vi "CPP_WhiteNoiseGenerator.vi"() -> ()   [LabVIEW 2012]
uses:
  <vilib>/sound2/lvsound2.llb/Sound Data Format.ctl
  <vilib>/sound2/lvsound2.llb/Sampling Mode.ctl
  <vilib>/Analysis/3filter.llb/Filter Passband Type.ctl
  Globals/Meas_global.vi
  Plug in sub vis/CPP_TubingCompensation/WhiteNoise/WhiteNoiseGlobal.vi
  <vilib>/Analysis/3filter.llb/Butterworth Filter (DBL).vi
  <vilib>/sound2/lvsound2.llb/Sound Output Write (DBL Single).vi
  <vilib>/measure/NI_MABase.lvlib
  <vilib>/Analysis/NI_AALBase.lvlib
panel:
  in  "Device ID":u32
  in  "Amplitude":dbl=1.0
  in  "Cutoff (Hz)":dbl=1000.0
  in  "Overproduce":dbl=1.2
  out "Duration (s)":dbl=16.0
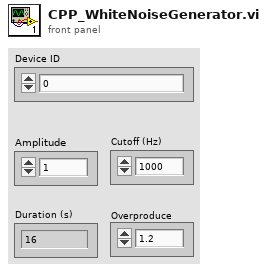
[diagram p1: front panel]
types:
  T1 = typedef "Post_Process.ctl" = enum16{"Take New Data", "Post Process Raw Data File"}
  T2 = typedef "NI_AALBase.lvlib/Filter Passband Type.ctl" = enum32{"Lowpass", "Highpass", "Bandpass", "Bandstop"}
  T3 = typedef "Sampling Mode.ctl" = i32
  T4 = typedef "Sound Data Format.ctl" = cluster{"sample rate (S/s)":dbl, "number of channels":i32, "bits per sample":i32}
  T5 = typedef "Sound Output Task ID.ctl" = u32
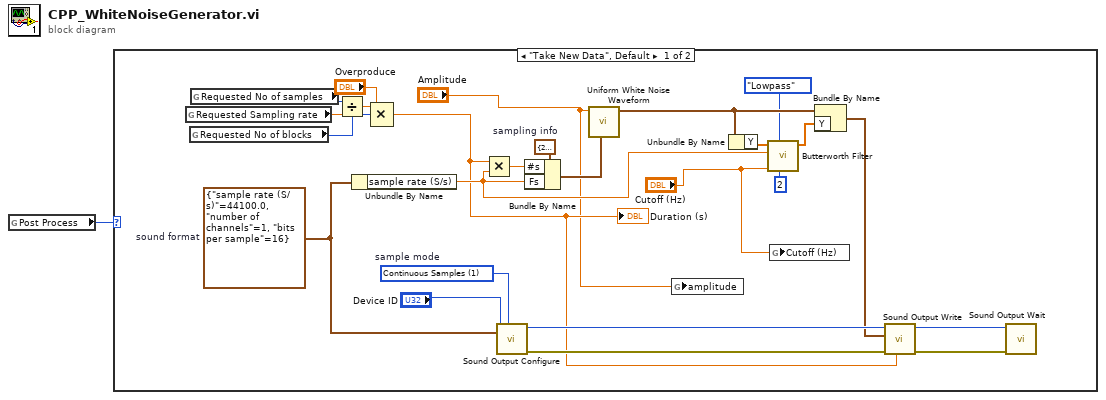
[diagram p0: block diagram]
diagram:
  n1 = global read "Meas_global.vi" "Post Process"() -> (w1:T1)
  n2 = case shown="\"Take New Data\", Default" w1 {
    frame "Take New Data", Default {
      w21 = T3 1 items=["Finite Samples", "Continuous Samples"]  # sample mode
      w23 = T4 {"sample rate (S/s)"=44100.0, "number of channels"=1, "bits per sample"=16}  # sound format
      w25 = cluster{"Fs":dbl, "#s":dbl} {"Fs"=22050.0, "#s"=22050.0}  # sampling info
      n3 = global read "Meas_global.vi" "Requested Sampling rate"() -> (w9:dbl)
      n4 = global read "Meas_global.vi" "Requested No of blocks"() -> (w7:i32)
      n5 = global read "Meas_global.vi" "Requested No of samples"() -> (w10:i32)
      n6 = Divide(x=w10, y=w9) -> (x/y=w8:dbl)
      n7 = Unbundle By Name(w23) -> ("sample rate (S/s)"=w15:dbl)
      n8 = Compound Arithmetic op=MULTIPLY(w8, w7, "Overproduce") -> (w5:dbl)
      "Duration (s)" <- w5
      n9 = Multiply(x=w5, y=w15) -> (x*y=w22:dbl)
      n10 = call <vilib>:"Sound Output Configure.vi"("sample mode"=w21, "sound format"=w23, "device ID"="Device ID") -> ("error out"=w26:errorcluster, "task ID"=w20:T5)  [unwired: 7 in]
      n11 = Bundle By Name(cluster=w25, "#s"=w22, "Fs"=w15) -> (w24:cluster{"Fs":dbl, "#s":dbl})
      n12 = call <vilib>:"Uniform White Noise Waveform.vi"("sampling info"=w24, "amplitude"="Amplitude") -> ("signal out"=w16:waveform(dbl))  [unwired: 8 in, 1 out]
      n13 = global write "WhiteNoiseGlobal.vi" "amplitude"("Amplitude") -> ()
      n14 = Unbundle By Name(w16) -> ("Y"=w13:dbl[])
      n15 = call-poly <vilib>:"Butterworth Filter.vi"("order"=2, "filter type"=Filter_Passband_Type."Lowpass", "low cutoff freq: fl"="Cutoff (Hz)", "sampling freq: fs"=w15, "X"=w13) -> ("Filtered X"=w17:dbl[])  [unwired: 3 in, 1 out]
      n16 = global write "WhiteNoiseGlobal.vi" "Cutoff (Hz)"("Cutoff (Hz)") -> ()
      n17 = Bundle By Name(cluster=w16, "Y"=w17) -> (w14:waveform(dbl))
      n18 = call-poly <vilib>:"Sound Output Write.vi"("timeout (sec)"=w5, "error in (no error)"=w26, "data"=w14, "task ID"=w20) -> ("error out"=w18:errorcluster, "task ID out"=w19:T5)  [unwired: 6 in]
      n19 = call <vilib>:"Sound Output Wait.vi"("error in (no error)"=w18, "task ID"=w19) -> ()  [unwired: 8 in, 2 out]
    }
    frame "Post Process Raw Data File" {
    }
  }
